vi "子VI-工件信息输入.vi"(8 "Y Resolution":i32, 9 "X Resolution":i32) -> (0 "质量等级":string, 1 "模式选择":u16(ring) items=["只读穿透图", "穿透图和反射图结合"], 3 "产品规格":cluster{"产品长度（周长）（mm）":dbl, "产品宽度（母线长）（mm）":dbl}, 4 "是否需要预处理":u16, 5 "图像分辨率":T1)   [LabVIEW 2018]
panel:
  in  "是否需要预处理（默认不进行预处理）":u16(ring) items=["需要预处理", "不需要预处理"]
  in  "模式选择":u16(ring) items=["只读穿透图", "穿透图和反射图结合"]
  in  "质量等级（请填入A/B/C，默认为B）":u16(ring) items=["A", "B", "C"]
  out "错误常量out":errorcluster
  in  "错误常量":errorcluster
  in  "停止按钮":bool
  in  "产品宽度（母线长）（mm）":dbl format="%#_13g"
  in  "产品长度（周长）（mm）":dbl format="%#_13g"
  in  "图像Y向分辨率（mm/像素）":dbl=1.0 format="%#_13g"
  in  "图像X向分辨率（mm/像素）":dbl=1.0 format="%#_13g"
  # "图像及工件参数输入"
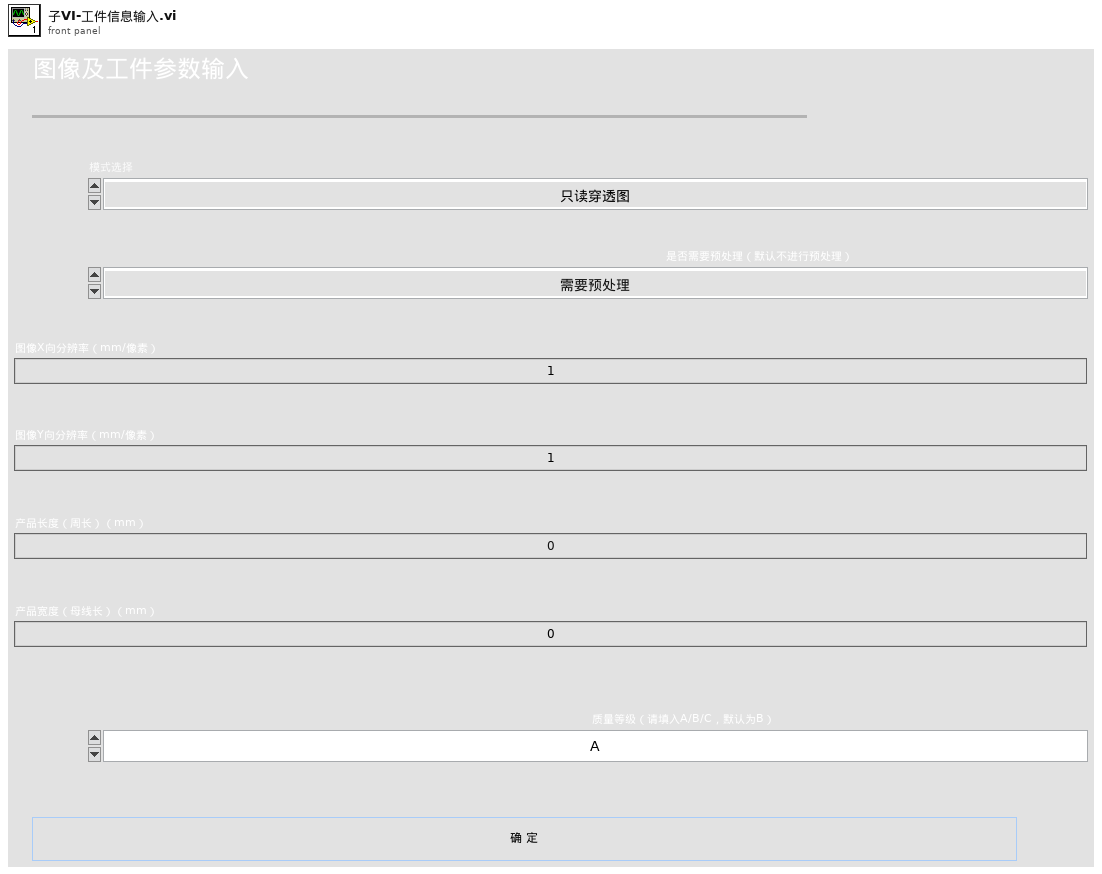
[diagram p1: front panel]
types:
  T1 = cluster{"图像X向分辨率（mm/像素）":dbl, "图像Y向分辨率（mm/像素）":dbl}
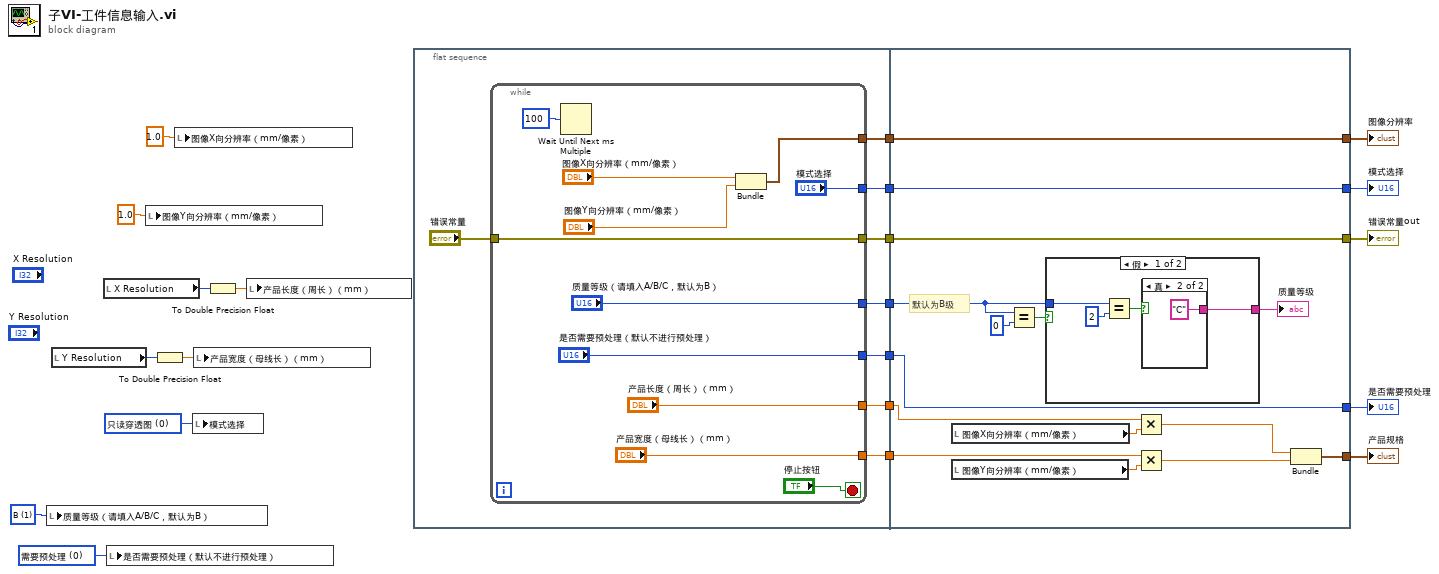
[diagram p0: block diagram]
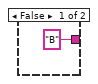
[diagram p2: hidden frame]
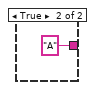
[diagram p3: hidden frame]
diagram:
  w9 = u16 0 items=["需要预处理", "不需要预处理"] ("是否需要预处理（默认不进行预处理）")
  w16 = u16 1 items=["A", "B", "C"] ("质量等级（请填入A/B/C，默认为B）")
  w17 = u16 0 items=["只读穿透图", "穿透图和反射图结合"] ("模式选择（默认只读穿透图）")
  n1 = local write "质量等级（请填入A/B/C，默认为B）"(w16) -> ()
  n2 = local read "Y Resolution"() -> (w13:i32)
  n3 = local read "X Resolution"() -> (w15:i32)
  n4 = local write "是否需要预处理（默认不进行预处理）"(w9) -> ()
  n5 = local write "图像Y向分辨率（mm/像素）"(1.0 ("图像Y向分辨率（mm/像素）")) -> ()
  n6 = To Double Precision Float(number=w13) -> (double precision float=w12:dbl)
  n7 = local write "图像X向分辨率（mm/像素）"(1.0 ("图像X向分辨率（mm/像素）")) -> ()
  n8 = local write "模式选择"(w17) -> ()
  n9 = local write "产品宽度（母线长）（mm）"(w12) -> ()
  n10 = To Double Precision Float(number=w15) -> (double precision float=w14:dbl)
  n11 = local write "产品长度（周长）（mm）"(w14) -> ()
  n12 = flat-sequence {
    tunnel: [w29] -> w8
    tunnel: [w28] -> w7
    tunnel: [w27] -> w6
    tunnel: [w26] -> w5
    tunnel: [w24] -> w4
    tunnel: [w23] -> w2
    tunnel: [w22] -> w1
    tunnel: [w53] -> w18
    tunnel: [w54] -> w19
    tunnel: [w47] -> w20
    tunnel: [w55] -> w21
    tunnel: w8 -> [w55]
    tunnel: w7 -> [w54]
    tunnel: w6 -> [w53]
    tunnel: w5 -> [w50]
    tunnel: w4 -> [w48]
    tunnel: [w48] -> w3
    tunnel: w2 -> [w46]
    tunnel: w1 -> [w42]
    frame #0 {
      n13 = while {
        tunnel: [w40] -> w29
        tunnel: "错误常量" -> [w36]
        tunnel: [w36] -> w28
        tunnel: ["质量等级（请填入A/B/C，默认为B）"] -> w26
        tunnel: ["模式选择"] -> w27
        tunnel: ["是否需要预处理（默认不进行预处理）"] -> w24
        tunnel: ["产品长度（周长）（mm）"] -> w23
        tunnel: ["产品宽度（母线长）（mm）"] -> w22
        stop <- "停止按钮" stop-if-true
        n14 = Wait Until Next ms Multiple(millisecond multiple=u32 100 ("毫秒倍数")) -> ()  [unwired: 1 out]
        n15 = Bundle("图像X向分辨率（mm/像素）"="图像X向分辨率（mm/像素）", "图像Y向分辨率（mm/像素）"="图像Y向分辨率（mm/像素）") -> (w40:T1)  [unwired: 1 in]
      }
    }
    frame #1 {
      # "默认为B级"
      n16 = local read "图像X向分辨率（mm/像素）"() -> (w45:dbl)
      n17 = local read "图像Y向分辨率（mm/像素）"() -> (w41:dbl)
      n18 = Equal?(x=w50, y=u16 0) -> (x = y?=w51:bool)
      n19 = case shown="假" w51 {
        tunnel: [w56 "A" ("质量等级")] -> w52
        tunnel: w50 -> [w58 _]
        frame False {
          n20 = Equal?(x=w58, y=u16 2) -> (x = y?=w57:bool)
          n21 = case shown="真" w57 {
            tunnel: ["B" ("质量等级") "C" ("质量等级")] -> w56
            frame False {
            }
            frame True {
            }
          }
        }
        frame True {
        }
      }
      "质量等级" <- w52
      n22 = Multiply(x=w46, y=w45) -> (x*y=w44:dbl)
      n23 = Multiply(x=w42, y=w41) -> (x*y=w43:dbl)
      n24 = Bundle(w44, w43) -> (w47:cluster{dbl, dbl})  [unwired: 1 in]
    }
  }
  "图像分辨率" <- w21
  "产品规格" <- w20
  "错误常量out" <- w19
  "模式选择" <- w18
  "是否需要预处理" <- w3
